vi "send.vi"(0 "object in":refnum<class "serial_work.lvclass">, 1 "写入缓冲区":string, 5 "error in (no error)":errorcluster) -> (14 "object out":refnum<class "serial_work.lvclass">, 19 "error out":errorcluster)   [LabVIEW 2016, in "serial_work.lvclass"]
uses:
  serial_work.lvclass
  serial_work.lvclass/serial_work.ctl
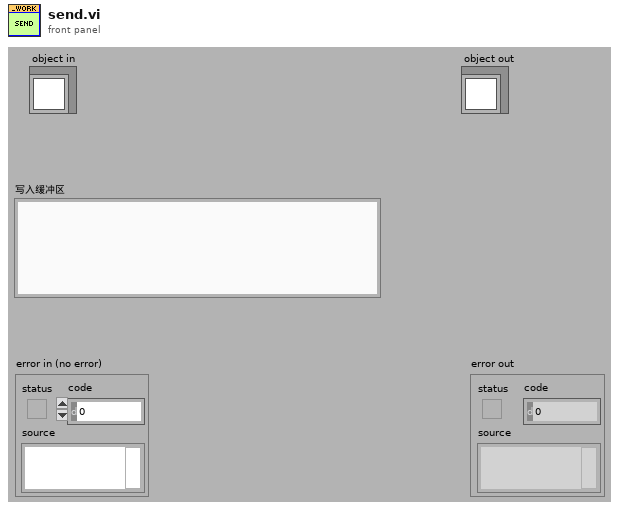
[diagram p1: front panel]
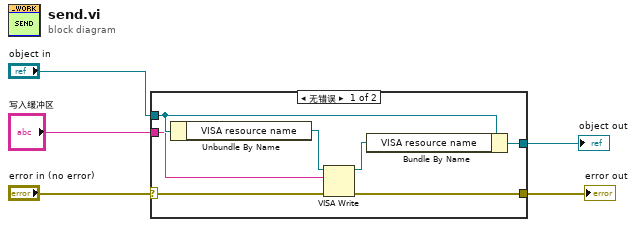
[diagram p0: block diagram]
diagram:
  n1 = case shown="无错误" "error in (no error)" {
    selector: "error in (no error)" -> [w7 w14]
    tunnel: [w6 w14] -> w4
    tunnel: [w11 w13] -> w2
    tunnel: "object in" -> [w12 w13]
    tunnel: "写入缓冲区" -> [w8 _]
    frame No Error {
      n2 = Unbundle By Name(w12) -> ("VISA resource name"=w10:refnum<visa-resource-name>)
      n3 = VISA Write(VISA resource name=w10, write buffer=w8, error in (no error)=w7) -> (VISA resource name out=w9:refnum<visa-resource-name>, error out=w6:errorcluster)  [unwired: 1 out]
      n4 = Bundle By Name(cluster=w12, "VISA resource name"=w9) -> (w11:refnum<class "serial_work.lvclass">)
    }
    frame Error {
    }
  }
  "error out" <- w4
  "object out" <- w2
